vi "Next Value - I32.vi"(8 "error in (no error)":errorcluster, 9 "timeout":dbl[unit]=1.0, 10 "default":i32, 11 "Subscription in":refnum<class "Subscription.lvclass">) -> (0 "error out":errorcluster, 1 "timed out?":bool, 2 "value":i32, 3 "Subscription out":refnum<class "Subscription.lvclass">, 4 "timestamp":timestamp, 5 "PV name":string)   [LabVIEW 2020, in "PV Access.lvlib" / "PVA Client.lvlib" / "Subscription.lvclass"]
uses:
  Subscription.lvclass
  Subscription.lvclass/Subscription.ctl
  53427cec-2bea-4028-8de6-3d4e850a6ab9.vi
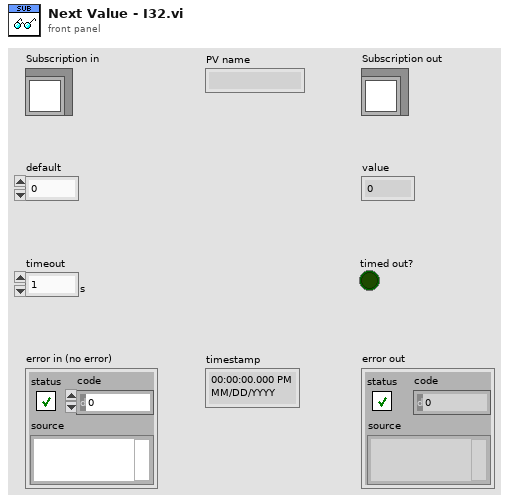
[diagram p1: front panel]
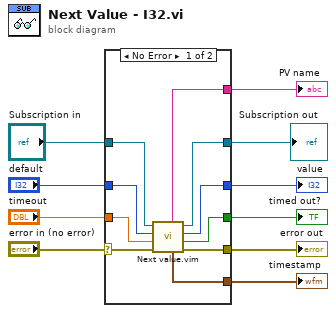
[diagram p0: block diagram]
diagram:
  n1 = case shown="No Error" "error in (no error)" {
    selector: "error in (no error)" -> [w18 w23]
    tunnel: [w17 w23] -> w9
    tunnel: [w19 w22] -> w7
    tunnel: "Subscription in" -> [w20 w22]
    tunnel: "timeout" -> [w16 _]
    tunnel: "default" -> [w15 w21]
    tunnel: [w14 w21] -> w4
    tunnel: [w13 _] -> w3
    tunnel: [w12 _] -> w2
    tunnel: [w11 _] -> w1
    frame No Error {
      n2 = call "Next value.vim"("error in"=w18, "timeout"=w16, "default"=w15, "Subscription in"=w20) -> ("error out"=w17:errorcluster, "timed out?"=w13:bool, "value"=w14:i32, "Subscription out"=w19:refnum<class "Subscription.lvclass">, "timestamp"=w11:timestamp, "PV name"=w12:string)  [unwired: 2 in]
    }
    frame Error {
    }
  }
  "error out" <- w9
  "Subscription out" <- w7
  "value" <- w4
  "timed out?" <- w3
  "PV name" <- w2
  "timestamp" <- w1
